vi "QueueToCommand.vi"(0 "ROS":T1={"topic port"=1236, "Node"="/labview", "topic"="/robot/head/command_head_nod", "type"="std_msgs/Bool", "node port"=7000, "error "={"status"=FALSE, "code"=0, "source"=""}, "Direction"=enum."Publisher", "Update (ms)"=1, "FIFO size"=1}, 2 "Check":enum16{"Cmd+FIFO", "FIFO", "CMD", "CMD /wait"}(ring)) -> (3 "ROS out":T1={"topic port"=1236, "Node"="/labview", "topic"="/robot/head/command_head_nod", "type"="std_msgs/Bool", "node port"=7000, "error "={"status"=FALSE, "code"=0, "source"=""}, "Direction"=enum."Publisher", "Update (ms)"=1, "FIFO size"=1}, 4 "Command":string, 5 "Queue log":string, 6 "data":string)   [LabVIEW 2012]
doc: "Executes a command from the queue"
uses:
  <userlib>/ROSforLV/ROS/Code/SubVIs/_ROSControl.ctl
  <userlib>/ROSforLV/ROS/Code/SubVIs/_ROSDirection.ctl
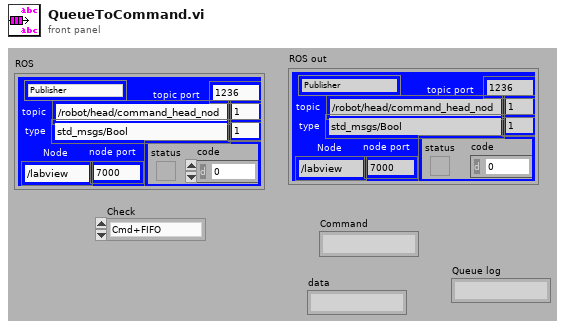
[diagram p1: front panel]
types:
  T1 = typedef "_ROSControl.ctl" = cluster{"topic port":u16, "Node":string, "topic":string, "type":string, "node port":u16, "error ":errorcluster, "Direction":T2, "Update (ms)":u16, "FIFO size":u16}
  T2 = typedef "_ROSDirection.ctl" = enum16{"Node", "Publisher", "Subscriber", "ServiceClient", "ServiceProvider"}
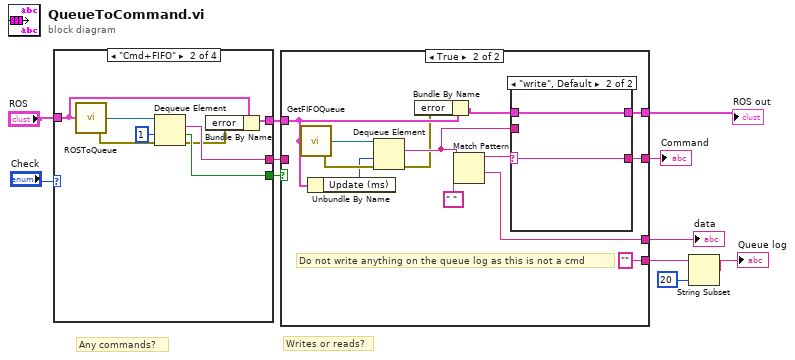
[diagram p0: block diagram]
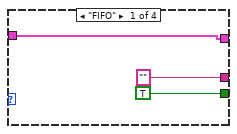
[diagram p2: hidden frame]
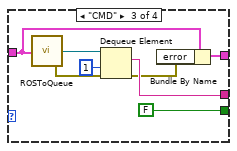
[diagram p3: hidden frame]
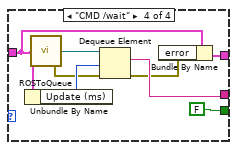
[diagram p4: hidden frame]
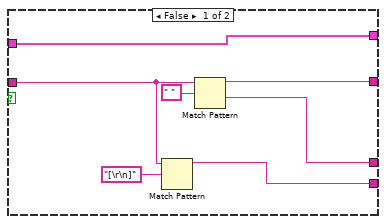
[diagram p5: hidden frame]
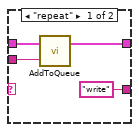
[diagram p6: hidden frame]
diagram:
  # "Writes or reads?"
  # "Any commands?"
  n1 = case shown="\"Cmd+FIFO\"" "Check" {
    tunnel: [TRUE ("timed out?") w20 FALSE ("timed out?") FALSE ("timed out?")] -> w11
    tunnel: "ROS" -> [w12 w17 w25 w33]
    tunnel: ["" w19 w29 w37] -> w8
    tunnel: [w12 w16 w24 w32] -> w2
    frame "FIFO" {
    }
    frame "Cmd+FIFO" {
      n2 = call <userlib>:"ROSToQueue.vi"("ROS"=w17) -> ("error out"=w18:errorcluster, "queue"=w22:refnum<queue>)  [unwired: 3 in]
      n3 = Dequeue Element(queue=w22, timeout in ms (-1)=1, error in (no error)=w18) -> (element=w19:string, timed out?=w20:bool, error out=w15:errorcluster)  [unwired: 1 out]
      n4 = Bundle By Name(cluster=w17, "error"=w15) -> (w16:T1)
    }
    frame "CMD" {
      n5 = call <userlib>:"ROSToQueue.vi"("ROS"=w25) -> ("error out"=w26:errorcluster, "queue"=w30:refnum<queue>)  [unwired: 3 in]
      n6 = Dequeue Element(queue=w30, timeout in ms (-1)=1, error in (no error)=w26) -> (element=w29:string, error out=w23:errorcluster)  [unwired: 2 out]
      n7 = Bundle By Name(cluster=w25, "error"=w23) -> (w24:T1)
    }
    frame "CMD /wait" {
      n8 = Unbundle By Name(w33) -> ("Update (ms)"=w35:u16)
      n9 = call <userlib>:"ROSToQueue.vi"("ROS"=w33) -> ("error out"=w34:errorcluster, "queue"=w38:refnum<queue>)  [unwired: 3 in]
      n10 = Dequeue Element(queue=w38, timeout in ms (-1)=w35, error in (no error)=w34) -> (element=w37:string, error out=w31:errorcluster)  [unwired: 2 out]
      n11 = Bundle By Name(cluster=w33, "error"=w31) -> (w32:T1)
    }
  }
  n12 = case shown="True" w11 {
    tunnel: [w41 w54] -> w10
    tunnel: [w40 ""] -> w6
    tunnel: [w42 w52] -> w9
    tunnel: w8 -> [w43 _]
    tunnel: w2 -> [w39 w50]
    tunnel: [w39 w48] -> w1
    frame False {
      n13 = Match Pattern(string=w43, regular expression="[\r\n]") -> (before substring=w40:string)  [unwired: 1 in, 3 out]
      n14 = Match Pattern(string=w43, regular expression=" ") -> (before substring=w42:string, after substring=w41:string)  [unwired: 1 in, 2 out]
    }
    frame True {
      # "Do not write anything on the queue log as this is not a cmd"
      n15 = call <userlib>:"GetFIFOQueue.vi"("ROS"=w50) -> ("error out"=w57:errorcluster, "queue out"=w58:refnum<queue>)  [unwired: 3 in]
      n16 = Unbundle By Name(w50) -> ("Update (ms)"=w56:u16)
      n17 = Dequeue Element(queue=w58, timeout in ms (-1)=w56, error in (no error)=w57) -> (element=w51:string, error out=w47:errorcluster)  [unwired: 2 out]
      n18 = Bundle By Name(cluster=w50, "error"=w47) -> (w49:T1)
      n19 = Match Pattern(string=w51, regular expression=" ") -> (before substring=w53:string, after substring=w54:string)  [unwired: 1 in, 2 out]
      n20 = case shown="\"write\", Default" w53 {
        selector: w53 -> [_ w64]
        tunnel: ["write" w64] -> w52
        tunnel: w49 -> [w61 w63]
        tunnel: w51 -> [w60 _]
        tunnel: [w59 w63] -> w48
        frame "repeat" {
          n21 = call <userlib>:"AddToQueue.vi"("Cmd"=w60, "ROS"=w61) -> ("ROS out"=w59:T1)  [unwired: 3 in]
        }
        frame "write", Default {
        }
      }
    }
  }
  "Command" <- w9
  "data" <- w10
  "ROS out" <- w1
  n22 = String Subset(string=w6, length (rest)=20 ("length (rest)")) -> (substring=→"Queue log":string)  [unwired: 1 in]
